vi "CODMnMB_api.vi"(6 "Slave ID":u8=1, 7 "STEP":enum16{"open", "read", "write", "close"}(ring)=enum."read", 8 "Error in":errorcluster caption="Error in (no error)", 9 "values":u16[](array[numeric]), 10 "quantity":u16, 11 "starting address":u16 format="%04xH") -> (0 "error out":errorcluster, 1 "MB session out":refnum<class "MB_Master.lvclass">, 2 "输出簇":T1, 3 "Registers":u16[](array[numeric]))   [LabVIEW 2016, in "斯坦道CODMn.lvlib"]
uses:
  <vilib>/Plasmionique/MB Master/MB_Master/MB_Master.lvclass
  <vilib>/Plasmionique/MB Master/MB_ADU/MB_ADU.lvclass/MB_ADU.ctl
  <vilib>/Plasmionique/MB Master/MB_ADU/Read RX Data.vi
  <vilib>/Plasmionique/MB Master/MB_ADU/Read RX Timestamp.vi
  <vilib>/Plasmionique/MB Master/MB_ADU/Read Slave ID.vi
  <vilib>/Plasmionique/MB Master/MB_ADU/Read TX Data.vi
  <vilib>/Plasmionique/MB Master/MB_ADU/Read TX Timestamp.vi
  <vilib>/Plasmionique/MB Master/MB_Master_Serial/MB_Master_Serial.lvclass
  C:/Program Files (x86)/National Instruments/LabVIEW 2016/vi.lib/Plasmionique/MB Master/MB_Master/MB_Master.lvclass
  <vilib>/Plasmionique/MB Master/MB_ADU/MB_ADU.lvclass
  <vilib>/Plasmionique/MB Master/MB Master.lvlib
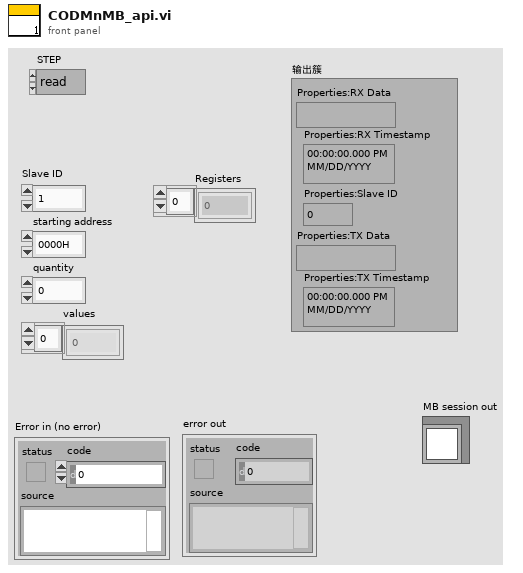
[diagram p1: front panel]
types:
  T1 = cluster{"Properties:RX Data":string, "Properties:RX Timestamp":timestamp, "Properties:Slave ID":u8, "Properties:TX Data":string, "Properties:TX Timestamp":timestamp}
  T2 = cluster{"baud rate (bps)":u32, "stop bits":u16, "parity":u16, "flow control":u16, "timeout":u32, "retries":i32}
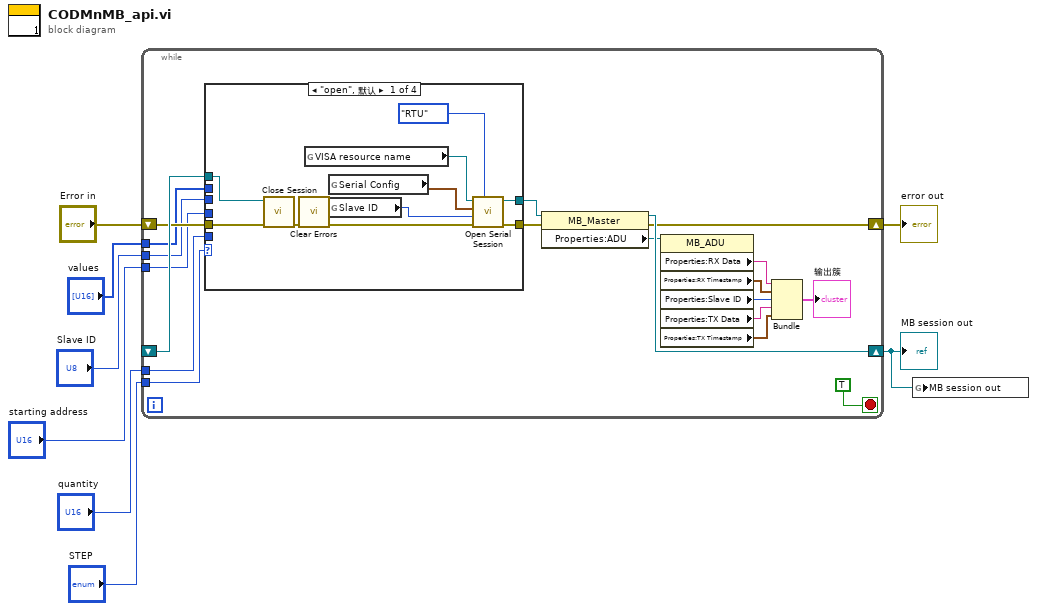
[diagram p0: block diagram]
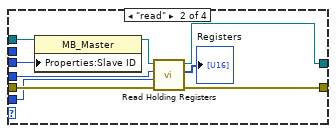
[diagram p2: hidden frame]
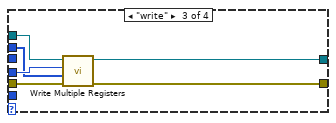
[diagram p3: hidden frame]
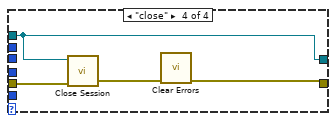
[diagram p4: hidden frame]
diagram:
  n1 = while {
    shift-right: [w21] -> w1
    shift-left: _ -> [w27]
    shift-right: [w19] -> w7
    shift-left: "Error in" -> [w26]
    tunnel: "Slave ID" -> [w25]
    tunnel: "starting address" -> [w24]
    tunnel: "quantity" -> [w23]
    tunnel: "STEP" -> [w22]
    tunnel: "values" -> [w11]
    stop <- TRUE stop-if-true
    n2 = case shown="\"open\", 默认" w22 {
      tunnel: w27 -> [w34 w39 w50 w55]
      tunnel: w26 -> [w33 w46 w52 w56]
      tunnel: [w35 w45 w49 w55] -> w9
      tunnel: [w36 w44 w51 w53] -> w20
      tunnel: w25 -> [_ w42 _ _]
      tunnel: w24 -> [_ w41 w48 _]
      tunnel: w23 -> [_ w40 _ _]
      tunnel: w11 -> [_ _ w47 _]
      frame "open", Default {
        n3 = call-dynamic "Close Session.vi"("error in (no error)"=w33, "MB session in"=w34) -> ("error out"=w32:errorcluster)  [unwired: 9 in]
        n4 = call <vilib>:"Clear Errors.vi"("error in (no error)"=w32) -> ("error out"=w28:errorcluster)  [unwired: 5 in, 1 out]
        n5 = global read "CODMn断电保存全局变量.vi" "VISA resource name"() -> (w31:refnum<visa-resource-name>)
        n6 = global read "CODMn断电保存全局变量.vi" "Serial Config"() -> (w29:T2)
        n7 = global read "CODMn断电保存全局变量.vi" "Slave ID"() -> (w30:u8)
        n8 = call <vilib>:"Open Serial Session.vi"("Mode (RTU)"=enum16{"RTU", "ASCII"}."RTU", "Error in"=w28, "Slave ID"=w30, "Serial Config"=w29, "VISA Resource"=w31) -> ("Error out"=w36:errorcluster, "MB_Serial session"=w35:refnum<class "MB_Master_Serial.lvclass">)  [unwired: 5 in]
      }
      frame "read" {
        n9 = property class="MB_Master"(reference=w39, "Properties:Slave ID"=w42) -> (reference out=w38:refnum<class "MB_Master.lvclass">)  [unwired: 1 in, 1 out]
        n10 = call <vilib>:"Read Holding Registers.vi"("error in (no error)"=w46, "quantity"=w40, "starting address"=w41, "MB session in"=w38) -> ("error out"=w44:errorcluster, "Registers"=→"Registers":u16[], "MB session out"=w45:refnum<class "MB_Master.lvclass">)  [unwired: 5 in]
      }
      frame "write" {
        n11 = call <vilib>:"Write Multiple Registers.vi"("error in (no error)"=w52, "values"=w47, "starting address"=w48, "MB session in"=w50) -> ("error out"=w51:errorcluster, "MB session out"=w49:refnum<class "MB_Master.lvclass">)  [unwired: 6 in]
      }
      frame "close" {
        n12 = call-dynamic "Close Session.vi"("error in (no error)"=w56, "MB session in"=w55) -> ("error out"=w54:errorcluster)  [unwired: 9 in]
        n13 = call <vilib>:"Clear Errors.vi"("error in (no error)"=w54) -> ("error out"=w53:errorcluster)  [unwired: 5 in, 1 out]
      }
    }
    n14 = property class="MB_Master"(reference=w9, error in=w20) -> (reference out=w21:refnum<class "MB_Master.lvclass">, error out=w19:errorcluster, "Properties:ADU"=w18:refnum<class "MB_ADU.lvclass">)
    n15 = property class="MB_ADU"(reference=w18) -> ("Properties:RX Data"=w17:string, "Properties:RX Timestamp"=w16:timestamp, "Properties:Slave ID"=w15:u8, "Properties:TX Data"=w14:string, "Properties:TX Timestamp"=w13:timestamp)  [unwired: 1 in, 2 out]
    n16 = Bundle("Properties:RX Data"=w17, "Properties:RX Timestamp"=w16, "Properties:Slave ID"=w15, "Properties:TX Data"=w14, "Properties:TX Timestamp"=w13) -> (→"输出簇":T1)  [unwired: 1 in]
  }
  "error out" <- w7
  "MB session out" <- w1
  n17 = global write "CODMn断电保存全局变量.vi" "MB session out"(w1) -> ()
